vi "SendTcpSettingCommand.vi"(6 "機器番号":u8, 9 "SettingData":string, 10 "Setting File Path":path=path "Setting", 11 "アドレス":string) -> (1 "送信文字列":string, 2 "空?":bool, 3 "Send List Out":cluster{"Address":string, "Data":string}[](array[cluster]))   [LabVIEW 2021]
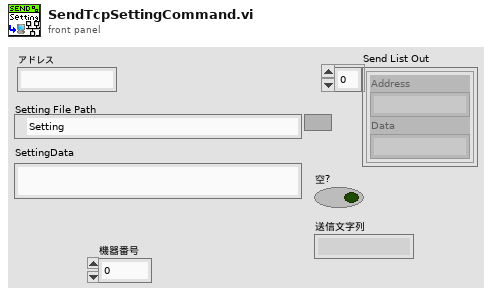
[diagram p1: front panel]
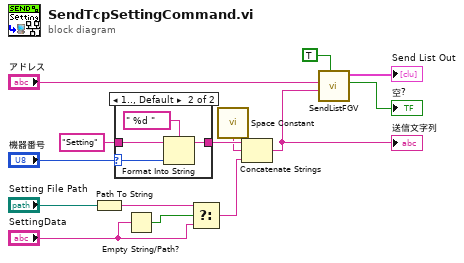
[diagram p0: block diagram]
diagram:
  n1 = Path To String(path="Setting File Path") -> (string=w2:string)
  n2 = case shown="1.., Default" "機器番号" {
    selector: "機器番号" -> [_ w17]
    tunnel: [w15 w19] -> w7
    tunnel: "Setting" ("要素") -> [w15 w16]
    frame 0 {
    }
    frame 1.., Default {
      n3 = Format Into String(format string=" %d " ("形式文字列"), initial string=w16, w17) -> (resulting string=w19:string)  [unwired: 1 in, 1 out]
    }
  }
  n4 = Empty String/Path?(string/path="SettingData") -> (empty?=w4:bool)
  n5 = Select(t=w2, s=w4, f="SettingData") -> (s? t:f=w1:string)
  n6 = call <vilib>:"Space Constant.vi"() -> ("String"=w5:string)
  n7 = Concatenate Strings(w7, w5, w1) -> (w6:string)
  "送信文字列" <- w6
  n8 = call "SendListFGV.vi"("Set"=TRUE, "Data"=w6, "アドレス"="アドレス") -> ("空?"=→"空?":bool, "Send List Out"=→"Send List Out":cluster{"Address":string, "Data":string}[])  [unwired: 6 in, 1 out]
